vi "deinit sync.vi"(8 "error in (no error)":errorcluster, 11 "Shared Memory runtime in":refnum<class "Shared Memory runtime.lvclass">) -> (0 "error out":errorcluster, 3 "Shared Memory runtime out":refnum<class "Shared Memory runtime.lvclass">)   [LabVIEW 2013, in "Shared Memory runtime.lvclass"]
uses:
  Shared Memory runtime.lvclass
  Shared Memory runtime.lvclass/Shared Memory runtime.ctl
  Read sync data.vi
  <vilib>/NI/Pthreads for LabVIEW on Linux RT/Classes/Semaphore/Semaphore.lvclass
  <vilib>/NI/Shared Memory Library/Classes/Shared Memory/Shared Memory.lvclass
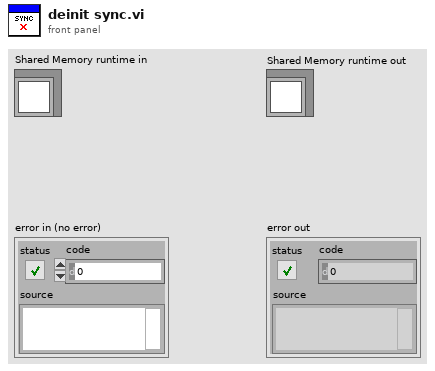
[diagram p1: front panel]
types:
  T1 = typedef "Shared Memory runtime.lvclass/sync data.ctl" = cluster{"semaphores soc":T2[], "semaphores eoc":T2[], "timeout":dbl, "enabled":bool, "sync shared memory":T4, "publish timing":bool, "timing indices":T5, "timing pointers":T6}
  T2 = typedef "Shared Memory runtime.lvclass/semaphore data.ctl" = cluster{"semaphore":T3, "name":string}
  T3 = typedef "POSIX Threads.lvlib/Semaphore.lvclass/reference.ctl" = refnum<data-value>
  T4 = typedef "Shared Memory.lvlib/Shared Memory.lvclass/reference.ctl" = refnum<data-value>
  T5 = typedef "Shared Memory runtime.lvclass/sync timing indices.ctl" = cluster{"start time index":i32}
  T6 = typedef "Shared Memory runtime.lvclass/sync timing pointers.ctl" = cluster{"start sec ptr":u64, "start nsec ptr":u64}
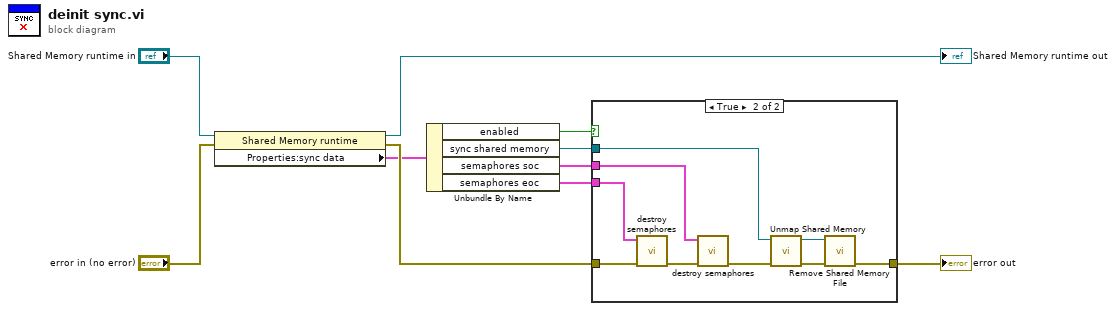
[diagram p0: block diagram]
diagram:
  n1 = property class="Shared Memory runtime"(reference="Shared Memory runtime in", error in="error in (no error)") -> (reference out=→"Shared Memory runtime out":refnum<class "Shared Memory runtime.lvclass">, error out=w8:errorcluster, "Properties:sync data"=w7:T1)
  n2 = Unbundle By Name(w7) -> ("enabled"=w5:bool, "sync shared memory"=w6:T4, "semaphores soc"=w2:T2[], "semaphores eoc"=w1:T2[])
  n3 = case shown="True" w5 {
    tunnel: [w11 w18] -> w9
    tunnel: w8 -> [w11 w16]
    tunnel: w6 -> [_ w17]
    tunnel: w2 -> [_ w12]
    tunnel: w1 -> [_ w13]
    frame False {
    }
    frame True {
      n4 = call "destroy semaphores.vi"("error in (no error)"=w16, "semaphores in"=w13) -> ("error out"=w15:errorcluster)  [unwired: 9 in]
      n5 = call "destroy semaphores.vi"("error in (no error)"=w15, "semaphores in"=w12) -> ("error out"=w14:errorcluster)  [unwired: 9 in]
      n6 = call <vilib>:"Unmap Shared Memory.vi"("error in (no error)"=w14, "shared memory in"=w17) -> ("error out"=w20:errorcluster, "shared memory out"=w19:T4)  [unwired: 8 in]
      n7 = call <vilib>:"Remove Shared Memory File.vi"("error in (no error)"=w20, "shared memory in"=w19) -> ("error out"=w18:errorcluster)  [unwired: 8 in, 1 out]
    }
  }
  "error out" <- w9
